vi "Toggle Laser.vi"(8 "Beam":bool, 11 "RS232":refnum<visa-resource-name>="ASRL27::INSTR") -> (0 "Success?":bool, 3 "RS232 out":refnum<visa-resource-name>="ASRL27::INSTR")   [LabVIEW 2022 SP3]
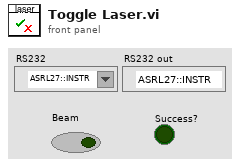
[diagram p1: front panel]
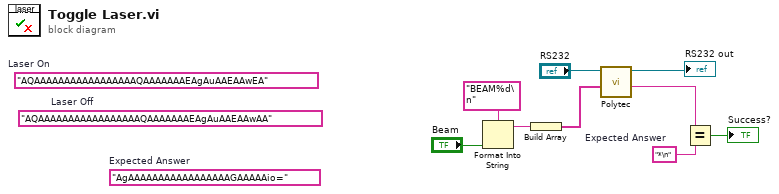
[diagram p0: block diagram]
diagram:
  w2 = "*\n"  # Expected Answer
  (unwired) "AQAAAAAAAAAAAAAAAAAQAAAAAAAEAgAuAAEAAwEA"  # Laser On
  (unwired) "AgAAAAAAAAAAAAAAAAAGAAAAAio="  # Expected Answer
  (unwired) "AQAAAAAAAAAAAAAAAAAQAAAAAAAEAgAuAAEAAwAA"  # Laser Off
  n1 = Format Into String(format string="BEAM%d\n", "Beam") -> (resulting string=w4:string)  [unwired: 2 in, 1 out]
  n2 = Build Array(w4) -> (w1:string[])
  n3 = call "Polytec.vi"("RS232"="RS232", "Strings"=w1) -> ("RS232 out"=→"RS232 out":refnum<visa-resource-name>, "String Read"=w3:string)  [unwired: 7 in]
  n4 = Equal?(x=w3, y=w2) -> (x = y?=→"Success?":bool)
